vi "Test Load Waveform from TDMS Backwards Compatibility.vi"(8 "error in (no error)":errorcluster) -> (0 "error out":errorcluster)   [LabVIEW 2016]
uses:
  <vilib>/addons/_JKI Toolkits/Caraya/classes/Assert/Assert Equal Value_Variant.vi
  <vilib>/addons/_JKI Toolkits/Caraya/classes/Assert/Assert Almost Equal_Float.vi
  Source/SG/SG.lvlib
  <vilib>/addons/_JKI Toolkits/Caraya/classes/Test/Test.lvclass
  <vilib>/addons/_JKI Toolkits/Caraya/classes/Assert/Assert.lvclass
  Source/Common/Common.lvlib
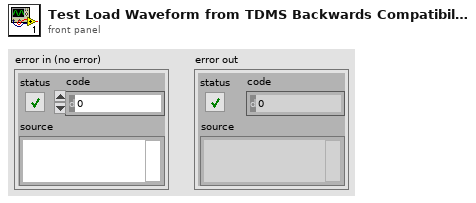
[diagram p1: front panel]
types:
  T1 = typedef "Common.lvlib/Waveform.ctl" = cluster{"Name":string, "Data":refnum<data-value>, "Signal Bandwidth (Hz)":dbl, "PAPR (dB)":dbl, "Burst Length (s)":dbl, "Sample Rate":dbl, "Burst Start Locations":i32[], "Burst Stop Locations":i32[], "Idle Duration Present?":bool, "Runtime Scaling":dbl, "Script":string}
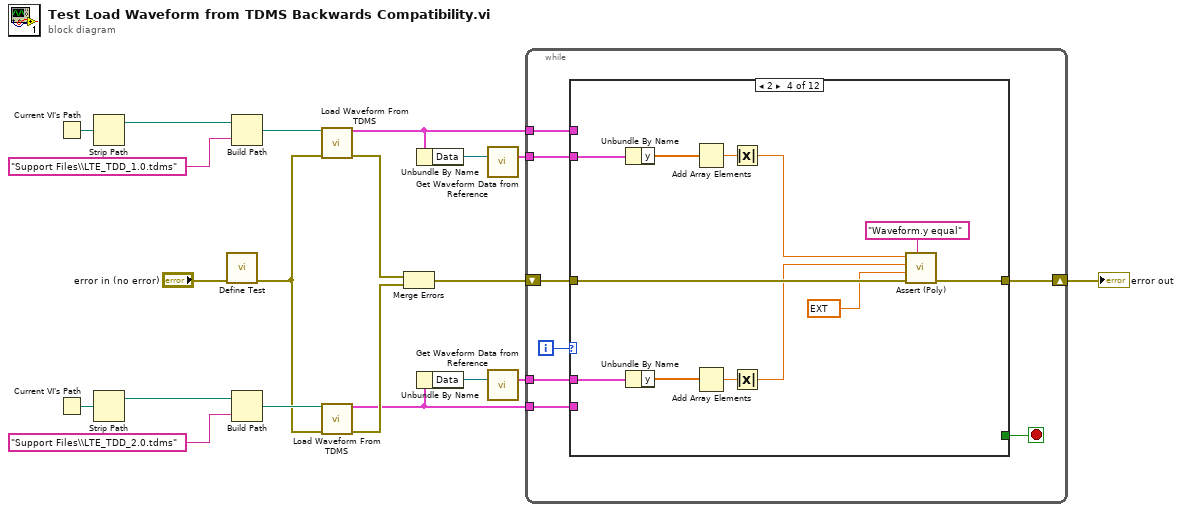
[diagram p0: block diagram]
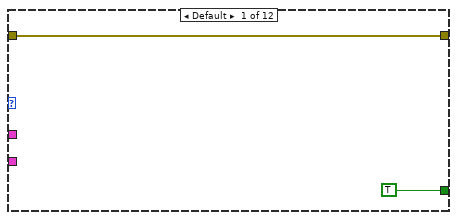
[diagram p2: hidden frame]
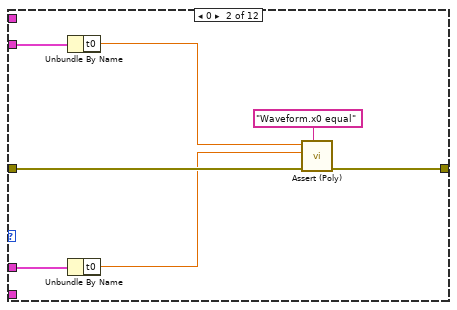
[diagram p3: hidden frame]
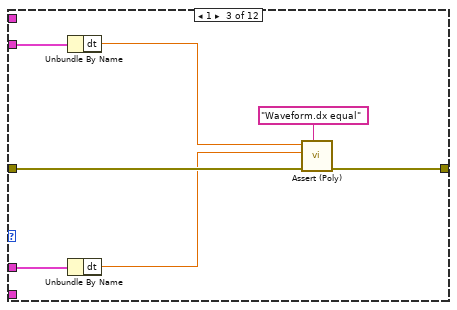
[diagram p4: hidden frame]
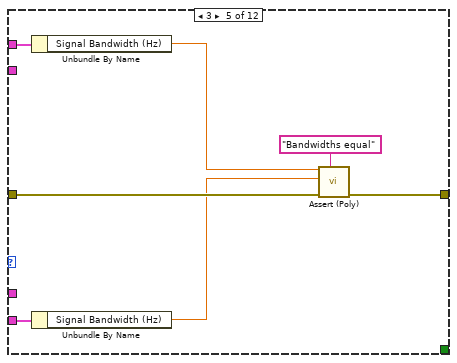
[diagram p5: hidden frame]
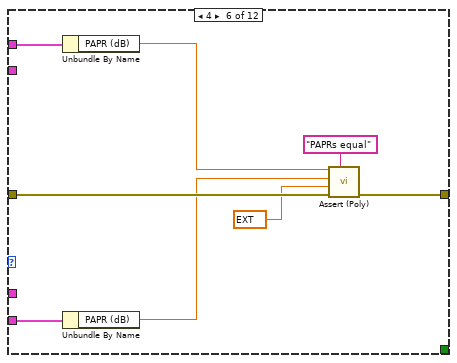
[diagram p6: hidden frame]
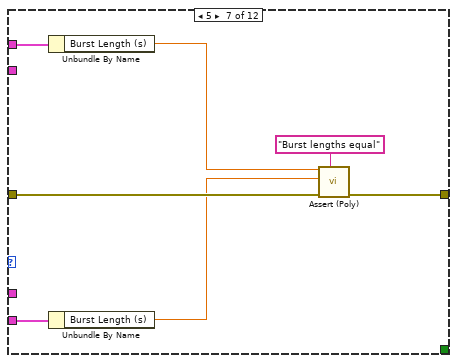
[diagram p7: hidden frame]
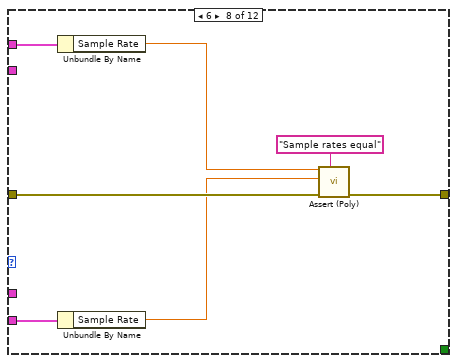
[diagram p8: hidden frame]
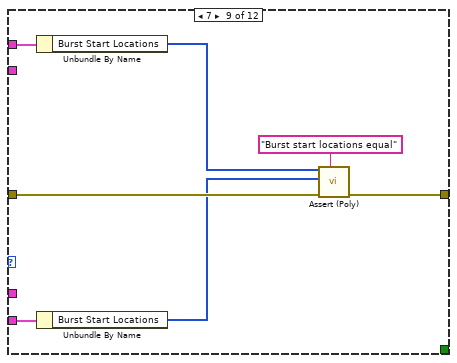
[diagram p9: hidden frame]
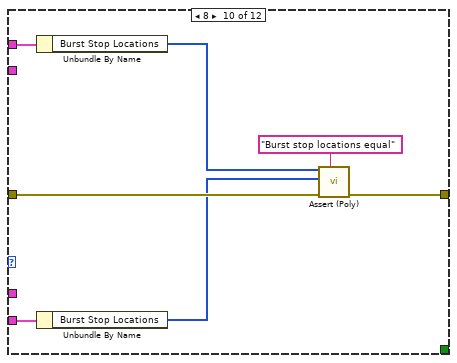
[diagram p10: hidden frame]
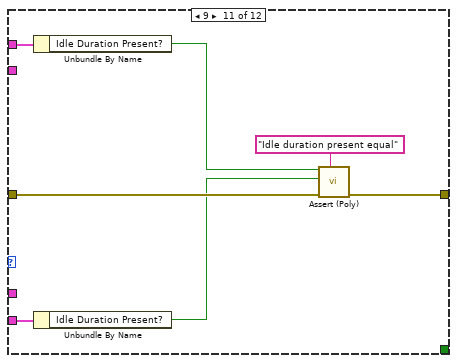
[diagram p11: hidden frame]
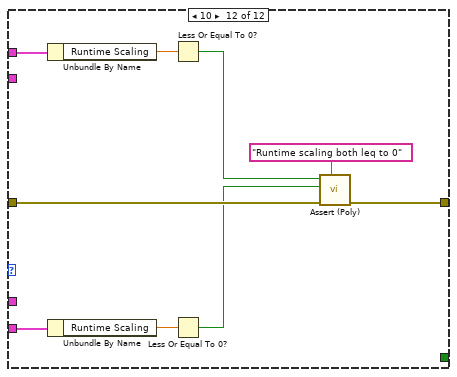
[diagram p12: hidden frame]
diagram:
  n1 = Current VI's Path() -> (path=w20:path)
  n2 = Current VI's Path() -> (path=w13:path)
  n3 = Strip Path(path=w20) -> (stripped path=w19:path)  [unwired: 1 out]
  n4 = Strip Path(path=w13) -> (stripped path=w14:path)  [unwired: 1 out]
  n5 = call <vilib>:"Define Test.vi"("error in (no error)"="error in (no error)") -> ("error out"=w11:errorcluster)  [unwired: 10 in]
  n6 = Build Path(base path=w19, name or relative path="Support Files\\LTE_TDD_1.0.tdms") -> (appended path=w17:path)
  n7 = Build Path(base path=w14, name or relative path="Support Files\\LTE_TDD_2.0.tdms") -> (appended path=w12:path)
  n8 = call "Load Waveform From TDMS.vi"("TDMS File Path"=w17, "error in (no error)"=w11) -> ("Waveform"=w6:T1, "error out"=w10:errorcluster)  [unwired: 12 in]
  n9 = call "Load Waveform From TDMS.vi"("TDMS File Path"=w12, "error in (no error)"=w11) -> ("Waveform"=w5:T1, "error out"=w9:errorcluster)  [unwired: 12 in]
  n10 = Merge Errors(w10, w9) -> (w8:errorcluster)
  n11 = Unbundle By Name(w6) -> ("Data"=w4:refnum<data-value>)
  n12 = Unbundle By Name(w5) -> ("Data"=w3:refnum<data-value>)
  n13 = call "Get Waveform Data from Reference.vi"("Waveform Data Reference"=w4) -> ("Waveform Data"=w2:cluster{"t0":dbl, "dt":dbl, "y":csg[]})  [unwired: 13 in, 1 out]
  n14 = call "Get Waveform Data from Reference.vi"("Waveform Data Reference"=w3) -> ("Waveform Data"=w1:cluster{"t0":dbl, "dt":dbl, "y":csg[]})  [unwired: 13 in, 1 out]
  n15 = while {
    shift-right: [w28] -> w7
    shift-left: w8 -> [w27]
    tunnel: w6 -> [w25]
    tunnel: w5 -> [w24]
    tunnel: w2 -> [w22]
    tunnel: w1 -> [w21]
    i -> [w26]
    stop <- w23 stop-if-true
    n16 = case shown="2" w26 {
      tunnel: [w29 w35 w42 w54 w61 w69 w76 w83 w90 w97 w104 w113] -> w28
      tunnel: w27 -> [w29 w36 w43 w55 w62 w70 w77 w84 w91 w98 w105 w114]
      tunnel: w25 -> [_ _ _ _ w60 w68 w75 w82 w89 w96 w103 w112]
      tunnel: w24 -> [_ _ _ _ w59 w67 w74 w81 w88 w95 w102 w111]
      tunnel: [TRUE _ _ _ _ _ _ _ _ _ _ _] -> w23
      tunnel: w22 -> [_ w32 w39 w46 _ _ _ _ _ _ _ _]
      tunnel: w21 -> [_ w31 w38 w45 _ _ _ _ _ _ _ _]
      frame Default {
      }
      frame 0 {
        n17 = Unbundle By Name(w32) -> ("t0"=w34:dbl)
        n18 = Unbundle By Name(w31) -> ("t0"=w33:dbl)
        n19 = call-poly <vilib>:"Assert (Poly).vi"("Label"="Waveform.x0 equal" ("format string"), "error in (no error)"=w36, "Y"=w33, "X"=w34) -> ("error out"=w35:errorcluster)  [unwired: 7 in]
      }
      frame 1 {
        n20 = Unbundle By Name(w39) -> ("dt"=w41:dbl)
        n21 = Unbundle By Name(w38) -> ("dt"=w40:dbl)
        n22 = call-poly <vilib>:"Assert (Poly).vi"("Label"="Waveform.dx equal" ("format string"), "error in (no error)"=w43, "Y"=w40, "X"=w41) -> ("error out"=w42:errorcluster)  [unwired: 7 in]
      }
      frame 2 {
        n23 = Unbundle By Name(w46) -> ("y"=w53:csg[])
        n24 = Unbundle By Name(w45) -> ("y"=w50:csg[])
        n25 = Add Array Elements(numeric array=w53) -> (sum=w52:csg)
        n26 = Add Array Elements(numeric array=w50) -> (sum=w51:csg)
        n27 = Absolute Value(x=w52) -> (abs(x)=w48:sgl)
        n28 = Absolute Value(x=w51) -> (abs(x)=w49:sgl)
        n29 = call-poly <vilib>:"Assert (Poly).vi"("Label"="Waveform.y equal" ("format string"), "error in (no error)"=w55, "Tolerance"=ext 0.00099999999999999999996, "Y"=w49, "X"=w48) -> ("error out"=w54:errorcluster)  [unwired: 6 in]
      }
      frame 3 {
        n30 = Unbundle By Name(w60) -> ("Signal Bandwidth (Hz)"=w58:dbl)
        n31 = Unbundle By Name(w59) -> ("Signal Bandwidth (Hz)"=w57:dbl)
        n32 = call-poly <vilib>:"Assert (Poly).vi"("Label"="Bandwidths equal" ("format string"), "error in (no error)"=w62, "Y"=w57, "X"=w58) -> ("error out"=w61:errorcluster)  [unwired: 7 in]
      }
      frame 4 {
        n33 = Unbundle By Name(w68) -> ("PAPR (dB)"=w66:dbl)
        n34 = Unbundle By Name(w67) -> ("PAPR (dB)"=w65:dbl)
        n35 = call-poly <vilib>:"Assert (Poly).vi"("Label"="PAPRs equal" ("format string"), "error in (no error)"=w70, "Tolerance"=ext 0.00099999999999999999996, "Y"=w65, "X"=w66) -> ("error out"=w69:errorcluster)  [unwired: 6 in]
      }
      frame 5 {
        n36 = Unbundle By Name(w75) -> ("Burst Length (s)"=w73:dbl)
        n37 = Unbundle By Name(w74) -> ("Burst Length (s)"=w72:dbl)
        n38 = call-poly <vilib>:"Assert (Poly).vi"("Label"="Burst lengths equal" ("format string"), "error in (no error)"=w77, "Y"=w72, "X"=w73) -> ("error out"=w76:errorcluster)  [unwired: 7 in]
      }
      frame 6 {
        n39 = Unbundle By Name(w82) -> ("Sample Rate"=w80:dbl)
        n40 = Unbundle By Name(w81) -> ("Sample Rate"=w79:dbl)
        n41 = call-poly <vilib>:"Assert (Poly).vi"("Label"="Sample rates equal" ("format string"), "error in (no error)"=w84, "Y"=w79, "X"=w80) -> ("error out"=w83:errorcluster)  [unwired: 7 in]
      }
      frame 7 {
        n42 = Unbundle By Name(w89) -> ("Burst Start Locations"=w87:i32[])
        n43 = Unbundle By Name(w88) -> ("Burst Start Locations"=w86:i32[])
        n44 = call-poly <vilib>:"Assert (Poly).vi"("Label"="Burst start locations equal" ("format string"), "error in (no error)"=w91, "Y"=w86, "X"=w87) -> ("error out"=w90:errorcluster)  [unwired: 7 in]
      }
      frame 8 {
        n45 = Unbundle By Name(w96) -> ("Burst Stop Locations"=w94:i32[])
        n46 = Unbundle By Name(w95) -> ("Burst Stop Locations"=w93:i32[])
        n47 = call-poly <vilib>:"Assert (Poly).vi"("Label"="Burst stop locations equal" ("format string"), "error in (no error)"=w98, "Y"=w93, "X"=w94) -> ("error out"=w97:errorcluster)  [unwired: 7 in]
      }
      frame 9 {
        n48 = Unbundle By Name(w103) -> ("Idle Duration Present?"=w101:bool)
        n49 = Unbundle By Name(w102) -> ("Idle Duration Present?"=w100:bool)
        n50 = call-poly <vilib>:"Assert (Poly).vi"("Label"="Idle duration present equal" ("format string"), "error in (no error)"=w105, "Y"=w100, "X"=w101) -> ("error out"=w104:errorcluster)  [unwired: 7 in]
      }
      frame 10 {
        n51 = Unbundle By Name(w112) -> ("Runtime Scaling"=w110:dbl)
        n52 = Unbundle By Name(w111) -> ("Runtime Scaling"=w109:dbl)
        n53 = Less Or Equal To 0?(x=w110) -> (x <= 0?=w108:bool)
        n54 = Less Or Equal To 0?(x=w109) -> (x <= 0?=w107:bool)
        n55 = call-poly <vilib>:"Assert (Poly).vi"("Label"="Runtime scaling both leq to 0" ("format string"), "error in (no error)"=w114, "Y"=w107, "X"=w108) -> ("error out"=w113:errorcluster)  [unwired: 7 in]
      }
    }
  }
  "error out" <- w7
